vi "Is Nominal State.vi"(11 "Base Actor in":refnum<class "Base Actor.lvclass">) -> (2 "Is Nominal State?":bool)   [LabVIEW 2021, in "jettl.lvlib" / "Actor.lvlib" / "Base Actor.lvclass"]
uses:
  Base Actor.lvclass
  State.ctl
  Base Actor.lvclass/Base Actor.ctl
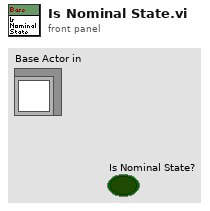
[diagram p1: front panel]
types:
  T1 = typedef "jettl.lvlib/Actor.lvlib/Base Actor.lvclass/State.ctl" = enum16{"Nominal", "Teardown", "Error"}
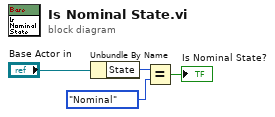
[diagram p0: block diagram]
diagram:
  n1 = Unbundle By Name("Base Actor in") -> ("State"=w2:T1)
  n2 = Equal?(x=w2, y=State."Nominal") -> (x = y?=→"Is Nominal State?":bool)
